vi "getAllActiveDevices.vi"(8 "error in (no error)":errorcluster, 11 "DeviceArray in":refnum<class "DeviceArray.lvclass">) -> (0 "error out":errorcluster, 2 "DeviceArray":refnum<class "DeviceArray.lvclass">, 3 "DeviceArray out":refnum<class "DeviceArray.lvclass">)   [LabVIEW 2009, in "Tools.lvlib" / "DatabaseHelpers.lvlib" / "DeviceArray.lvclass"]
uses:
  DeviceArray.lvclass
  device/device.lvclass
  DeviceArray.lvclass/DeviceArray.ctl
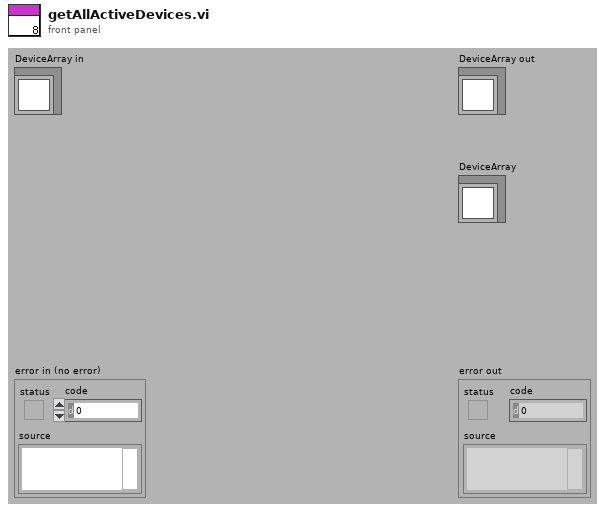
[diagram p1: front panel]
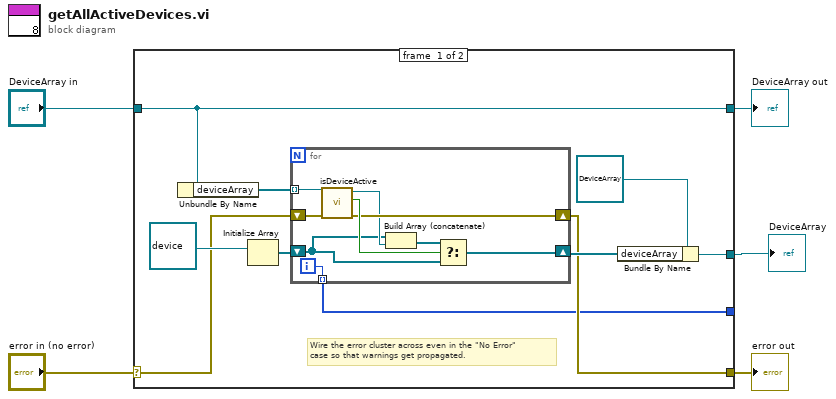
[diagram p0: block diagram]
diagram:
  n1 = case shown="No Error" "error in (no error)" {
    selector: "error in (no error)" -> [w8 w26]
    tunnel: [w7 w26] -> w4
    tunnel: [w13 w25] -> w2
    tunnel: "DeviceArray in" -> [w13 w25]
    tunnel: [w9 _] -> w1
    tunnel: [w6 _] -> _
    frame #0 {
      # "Wire the error cluster across even in the \"No Error\"\ncase so that warnings get propagated."
      n2 = Unbundle By Name(w13) -> ("deviceArray"=w15:refnum<class "device.lvclass">[])
      n3 = Initialize Array(refnum<class "device.lvclass"> refnum ("device out")) -> (w14:refnum<class "device.lvclass">[])  [unwired: 1 in]
      n4 = for {
        tunnel: w15 -> [w24] mode=indexing
        shift-right: [w21] -> w7
        shift-left: w8 -> [w23]
        shift-right: [w18] -> w10
        shift-left: w14 -> [w17]
        tunnel: [w16] -> w6 mode=indexing
        i -> [w16]
        n5 = call "isDeviceActive.vi"("error in (no error)"=w23, "device in"=w24) -> ("error out"=w21:errorcluster, "active"=w22:bool, "device out"=w20:refnum<class "device.lvclass">)  [unwired: 7 in]
        n6 = Build Array (concatenate)(w17, w20) -> (w19:refnum<class "device.lvclass">[])
        n7 = Select(t=w19, s=w22, f=w17) -> (s? t:f=w18:refnum<class "device.lvclass">[])
      }
      n8 = Bundle By Name(cluster=refnum<class "DeviceArray.lvclass"> refnum ("DeviceArray in"), "deviceArray"=w10) -> (w9:refnum<class "DeviceArray.lvclass">)
    }
    frame #1 {
    }
  }
  "error out" <- w4
  "DeviceArray out" <- w2
  "DeviceArray" <- w1
